vi "Process.vi"(8 "error in":errorcluster, 11 "IPS120":refnum<class "IPS120.lvclass">) -> (0 "error out":errorcluster, 3 "IPS120 out":refnum<class "IPS120.lvclass">)   [LabVIEW 2016, in "IPS120.lvclass"]
doc: "---------------------------------------------------------------\nJKI State Machine Objects™\nhttp://jki.net/state-machine-objects/\nCopyright (C) 2005-2015, JKI <info@jki.net>\nALL RIGHTS RESERVED"
uses:
  IPS120.lvclass
  IPS120/Typedefs/Read System 1 - Enum.ctl
  IPS120/Typedefs/Read System 2 - Enum.ctl
  IPS120/Typedefs/Read Activity - Enum.ctl
  IPS120/Typedefs/Read Switch Heater - Enum.ctl
  IPS120/Typedefs/Read Mode 1 - Enum.ctl
  IPS120/Typedefs/Read Mode 2 - Enum.ctl
  C:/Program Files (x86)/National Instruments/LabVIEW 2016/vi.lib/JKI/JKI SMO/SMO/SMO.lvclass
  <vilib>/JKI/JKI SMO/SMO/Typedefs/Parent Call--Enum.ctl
  <userlib>/LevyLab/Levylab Instruments/SMOs/Instrument/Instrument.lvclass
  <vilib>/JKI/JKI SMO/SMO/SMO.lvclass
  IPS-120.lvlib
panel:
  in  "Tab Control":enum32{"Front Panel", "Error Log"}(tab)
  out "Switch Message":string="Clamped"
  out "Persistent Field (T)":dbl=0.0001 format="%#.5f"
  out "PS Status":bool
  out "system status":T7={"System 1"=enum."Normal", "System 2"=enum."Outside Positive Current Limi", "Activity"=enum."Hold", "Switch Heater"=enum."No Switch Fitted", "Mode 1"=enum."Amps Fast", "Mode 2"=enum."At Rest"}
  out "Current (A)":dbl(knob)=0.0006 scale=-180.0..180.0
  out "Voltage (V) 2":dbl(knob)=-0.0003 caption="Voltage (V)" scale=-10.0..10.0
  out "Sentinel":bool=TRUE
  in  "Remote Mode":bool
  out "Power Supply Field (T)":dbl=0.0001 format="%#.5f"
  out "Voltage (V)":dbl=-0.0003 format="%.5f"
  out "PS Current (A)":dbl=0.0006 format="%.4f"
  out "Magnet Field (T)":dbl(knob) caption="Voltage (V)" scale=-20.0..20.0
  in  "Stop":bool
  out "Switch Time":string="11:11:48"
  in  "PS Heat":bool
  in  "Clamp":bool
  in  "To Set":bool
  in  "To Zero":bool
  in  "Hold":bool
  out "Magnet Activity":string="Clamped"
  out "Target Field Rate (T/min)":dbl=1.0 format="%.5f"
  out "Target Field (T) 2":dbl format="%#.5f"
  in  "Target Rate (T/min)":dbl=0.1 format="%.5f"
  in  "Target Field (T)":dbl format="%#.5f"
  in  "Send to IPS":bool
  out "Error List":T8(array[cluster])
  in  "IPS120 Address":refnum<visa-resource-name>="GPIB1::24::INSTR"
  # "For instructions on how to use the JKI State Machine Objects, examples and video tutorials, visit:\nhttp://jki.net/state-machine-objects/\n\nJKI State Machine Objects™\nhttp://jki.net/state-machine-objects/\nCopyright (C) 2005-2015, JKI <info@jki.net>\nALL RIGHTS RESERVED"
  # "System Status"
  # "Current (A)"
  # "Voltage (V)"
  # "Magnet (T)"
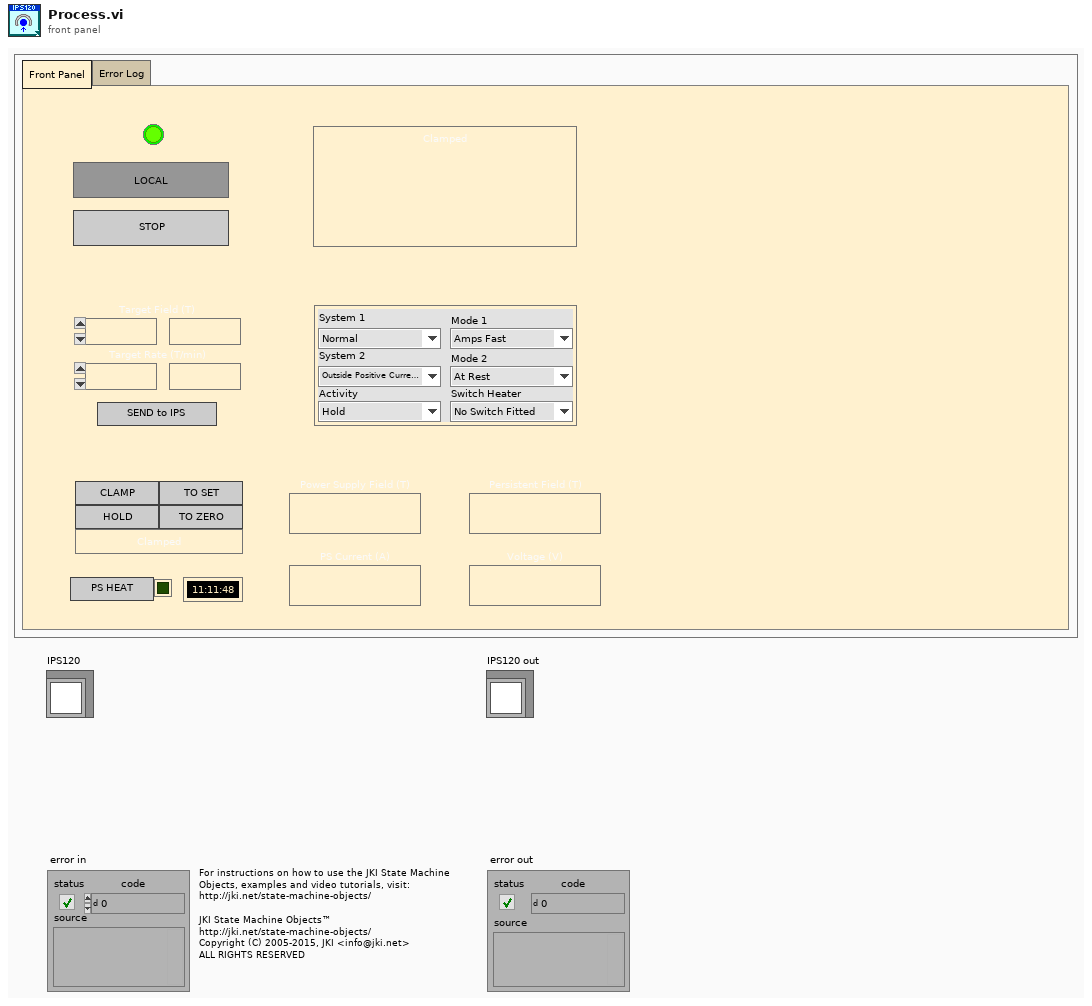
[diagram p1: front panel]
types:
  T1 = typedef "IPS-120.lvlib/Read System 1 - Enum.ctl" = enum16{"Normal", "Quenched", "Over Heated", "Warming Up", "Fault"}
  T2 = typedef "IPS-120.lvlib/Read System 2 - Enum.ctl" = enum16{"Normal", "On Positive Voltage Limit", "On Negative Voltage Limit", "Outside Negative Current Limit", "Outside Positive Current Limi"}
  T3 = typedef "IPS-120.lvlib/Read Activity - Enum.ctl" = enum16{"Hold", "To Set Point", "To Zero", "Clamped"}
  T4 = typedef "IPS-120.lvlib/Read Switch Heater - Enum.ctl" = enum16{"Off Magnet at Zero", "On", "Off Magnet at Field", "Heater Fault", "No Switch Fitted"}
  T5 = typedef "IPS-120.lvlib/Read Mode 1 - Enum.ctl" = enum16{"Amps Fast", "Tesla Fast", "Amps Slow", "Tesla Slow"}
  T6 = typedef "IPS-120.lvlib/Read Mode 2 - Enum.ctl" = enum16{"At Rest", "Sweeping", "Sweep Limiting", "Sweeping & Sweep Limiting"}
  T7 = cluster{"System 1":T1, "System 2":T2, "Activity":T3, "Switch Heater":T4, "Mode 1":T5, "Mode 2":T6}
  T8 = cluster{"time":timestamp, "code":i32, "source":string}[]
  T9 = typedef "SMO.lvclass/Parent Call--Enum.ctl" = enum16{"Allows parent to run", "Does not request parent to run"}
  T10 = enum32{"invalid app kind", "Development System", "Run Time System", "Student Edition", "Embedded LabVIEW", "Evaluation", "Custom"}
  T11 = enum32{"Invalid", "Standard", "Closed", "Hidden", "Minimized", "Maximized"}
  T12 = enum32{"Bad", "Idle", "Run top level", "Running"}
  T13 = cluster{"Core":cluster{"Current VI Reference":refnum<vi>, "Close Panel on Exit?":bool, "error":errorcluster}, "Self Reference":refnum<class "IPS120.lvclass">, "Your string data":string}
  T14 = cluster{"Current VI Reference":refnum<vi>, "Close Panel on Exit?":bool, "error":errorcluster}
  T15 = typedef "SMO.lvclass/Protected Events.ctl" = cluster{"StopProcesses":refnum<user-event>, "AbortProcesses":refnum<user-event>, "Config Changed":refnum<user-event>, "Dependency":refnum<user-event>}
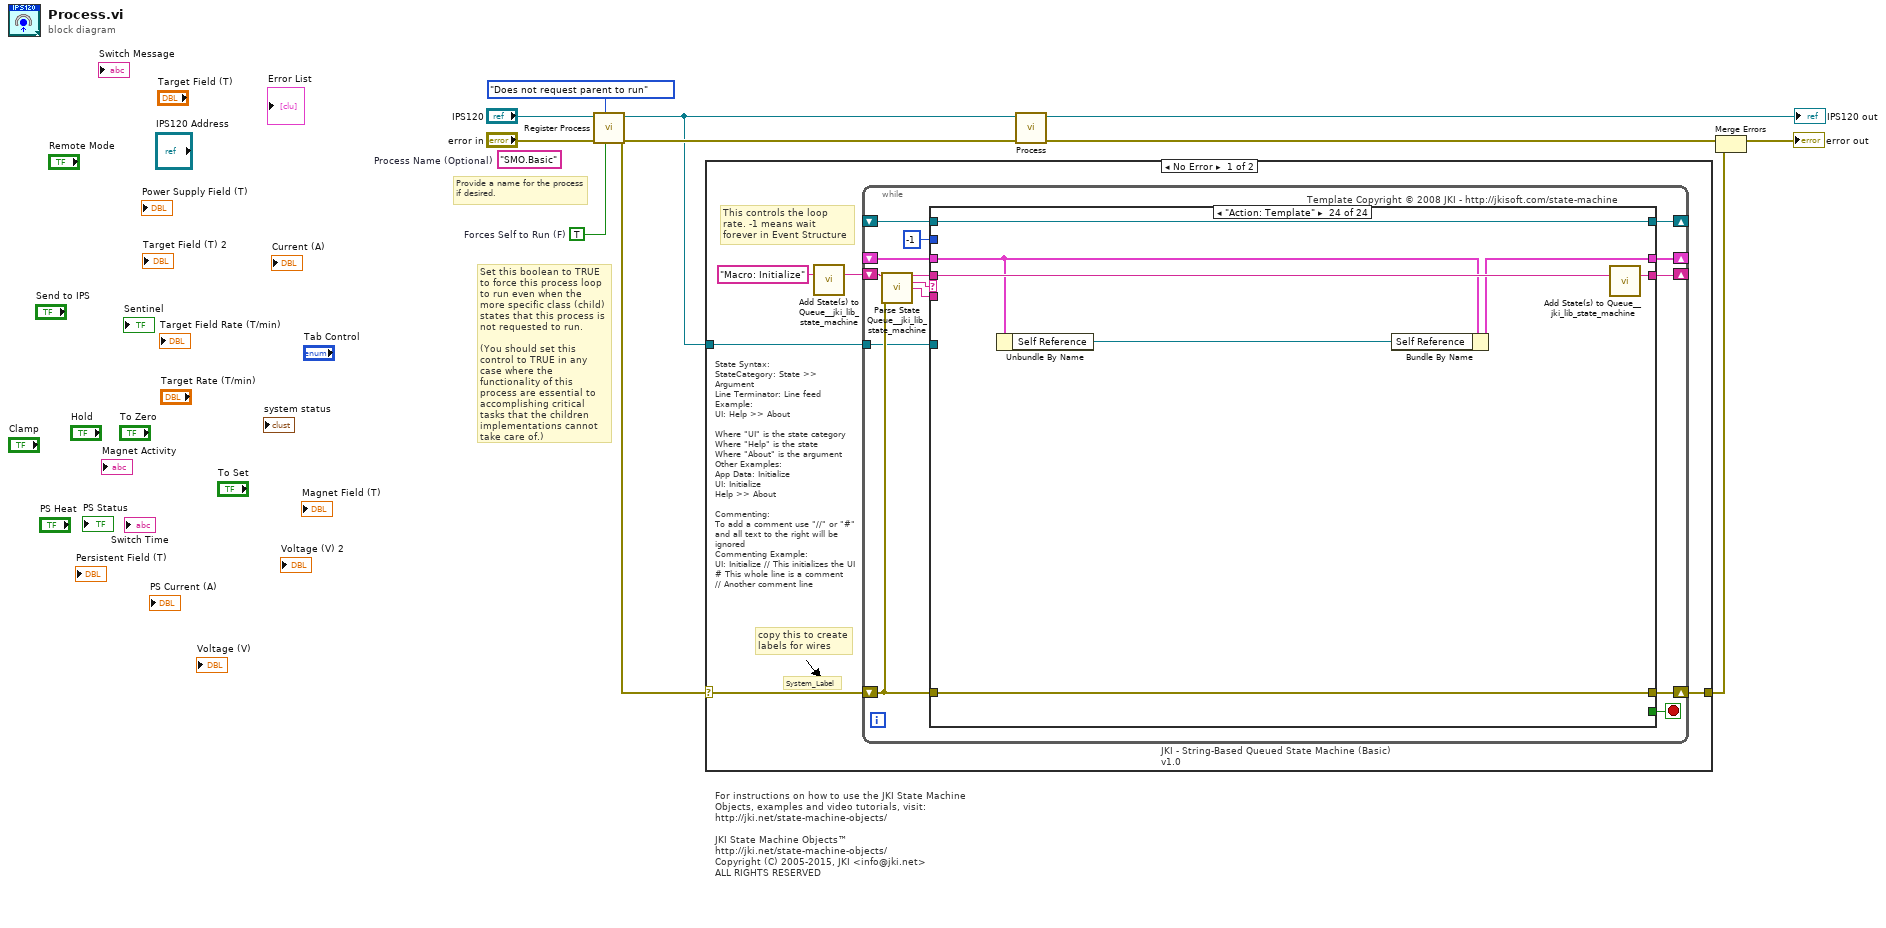
[diagram p0: block diagram]
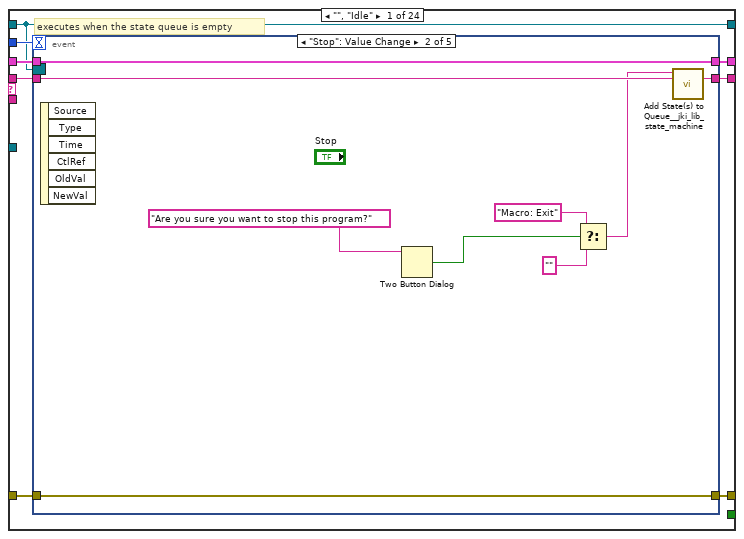
[diagram p2: hidden frame]
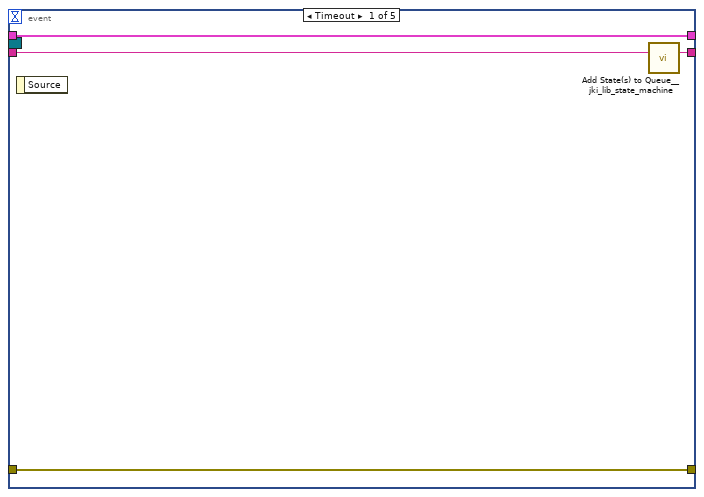
[diagram p3: hidden frame]
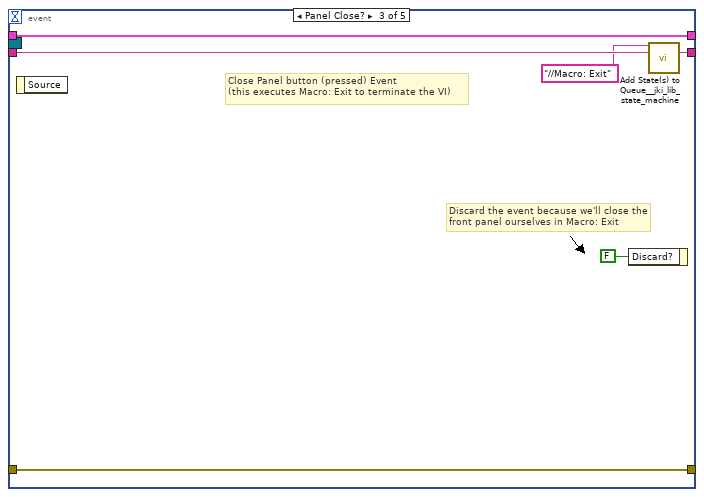
[diagram p4: hidden frame]
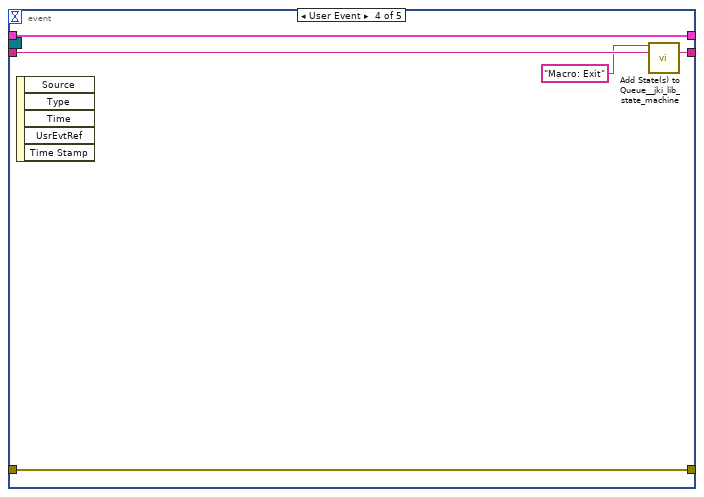
[diagram p5: hidden frame]
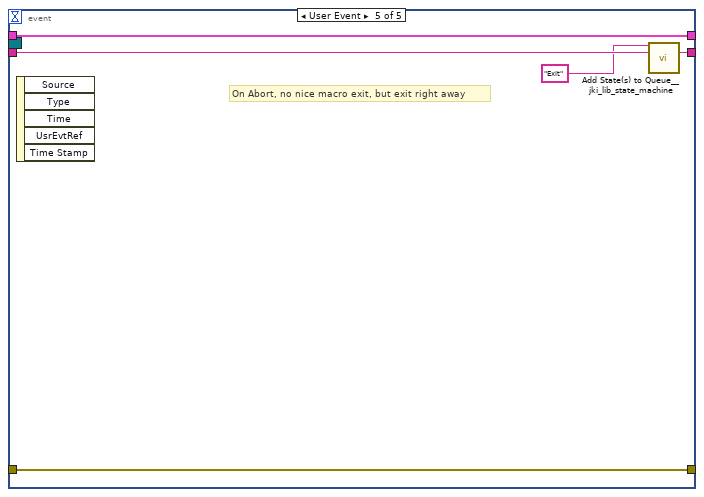
[diagram p6: hidden frame]
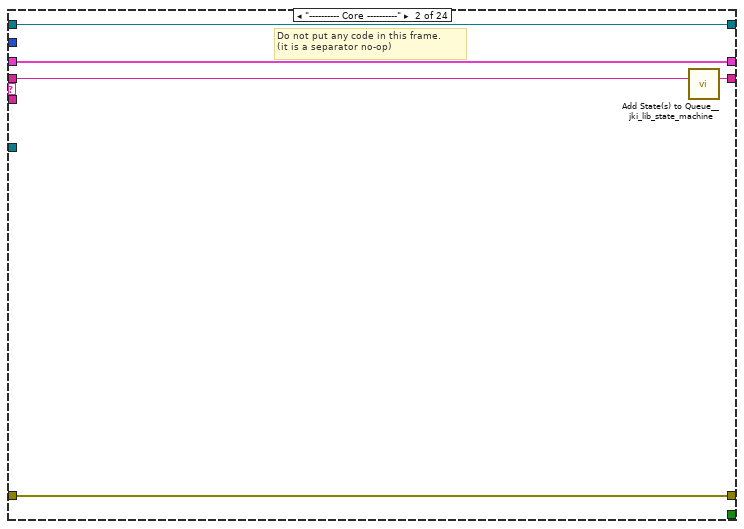
[diagram p7: hidden frame]
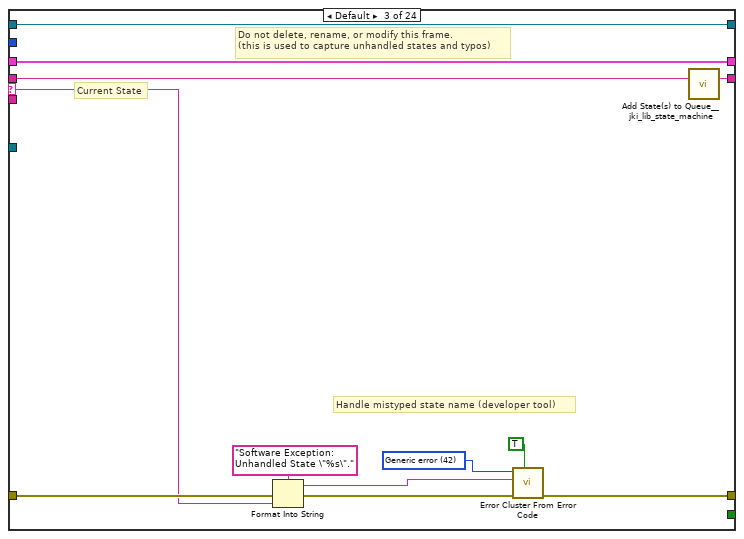
[diagram p8: hidden frame]
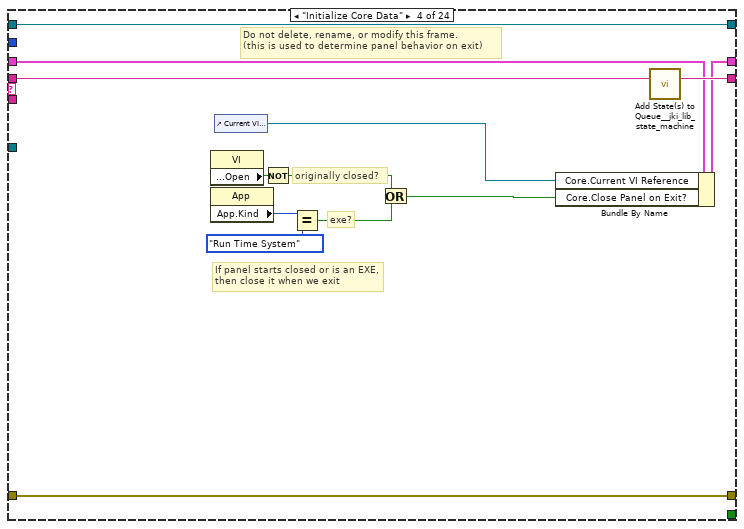
[diagram p9: hidden frame]
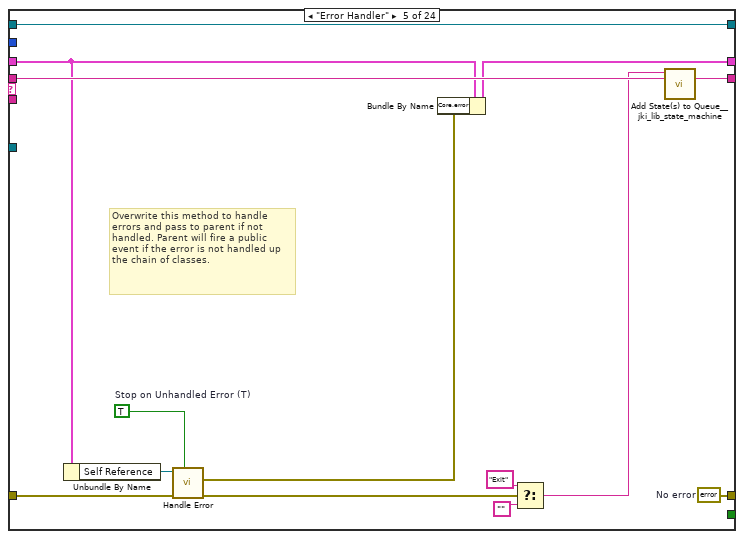
[diagram p10: hidden frame]
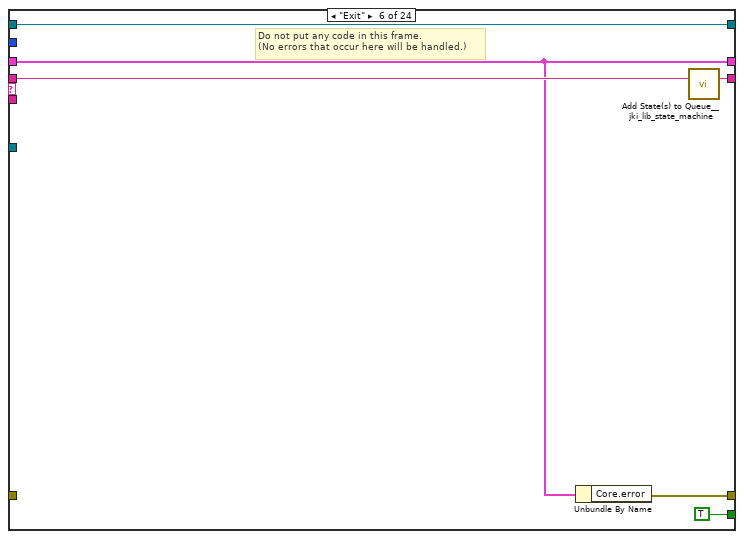
[diagram p11: hidden frame]
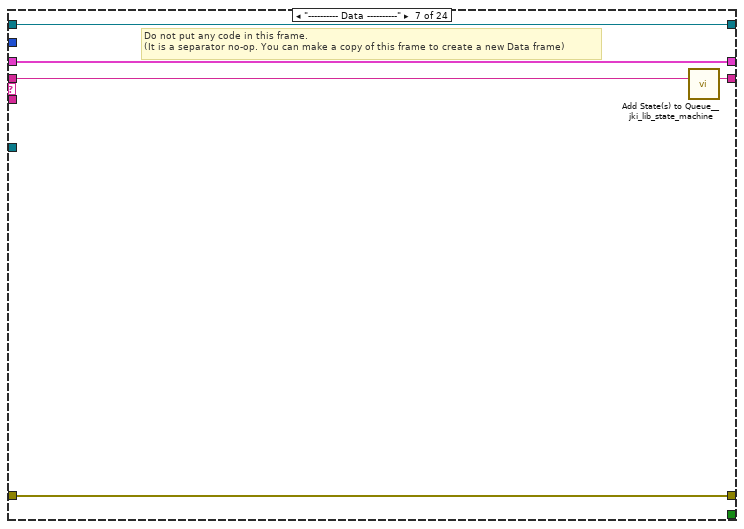
[diagram p12: hidden frame]
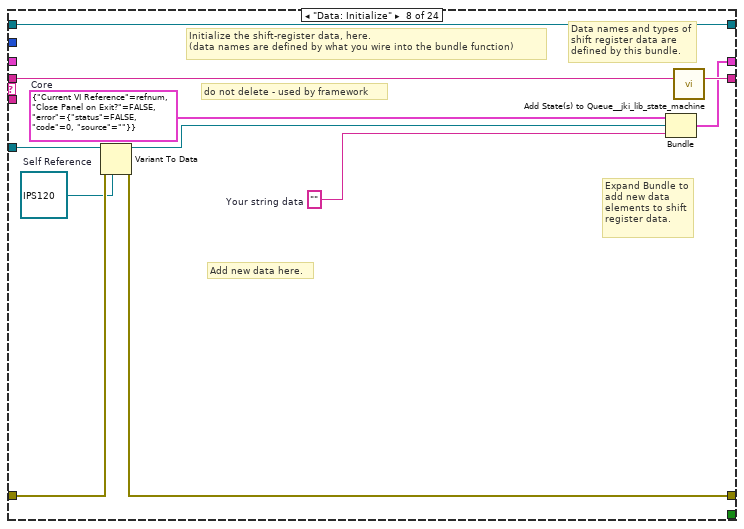
[diagram p13: hidden frame]
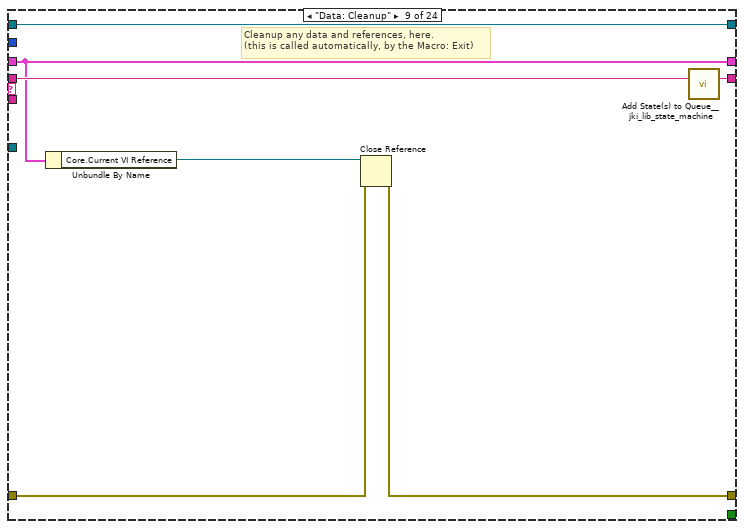
[diagram p14: hidden frame]
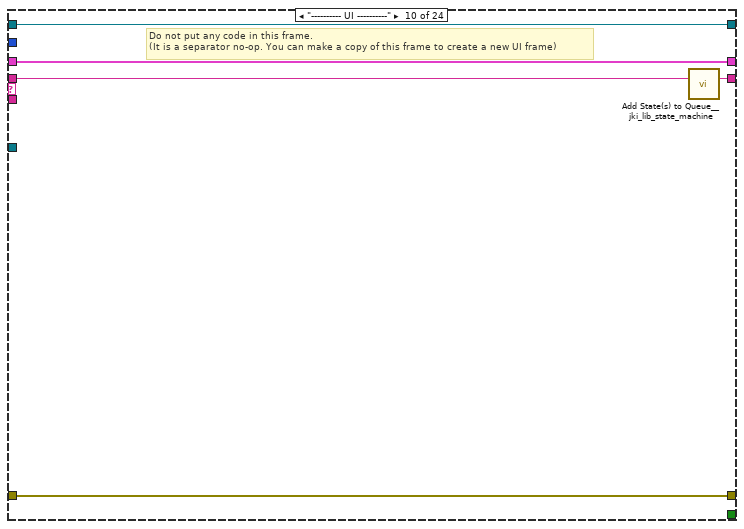
[diagram p15: hidden frame]
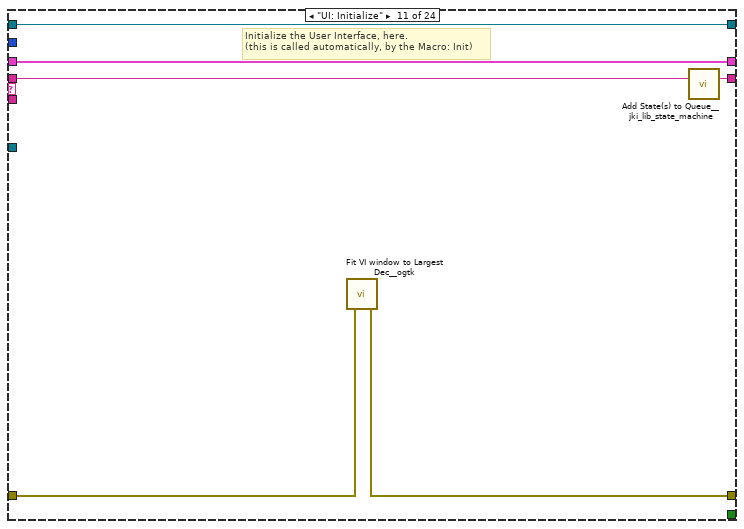
[diagram p16: hidden frame]
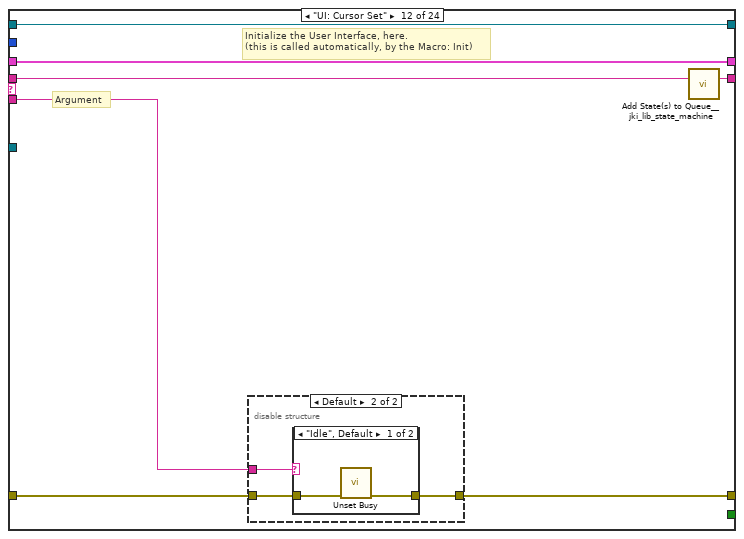
[diagram p17: hidden frame]
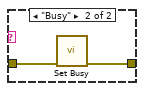
[diagram p19: hidden frame]
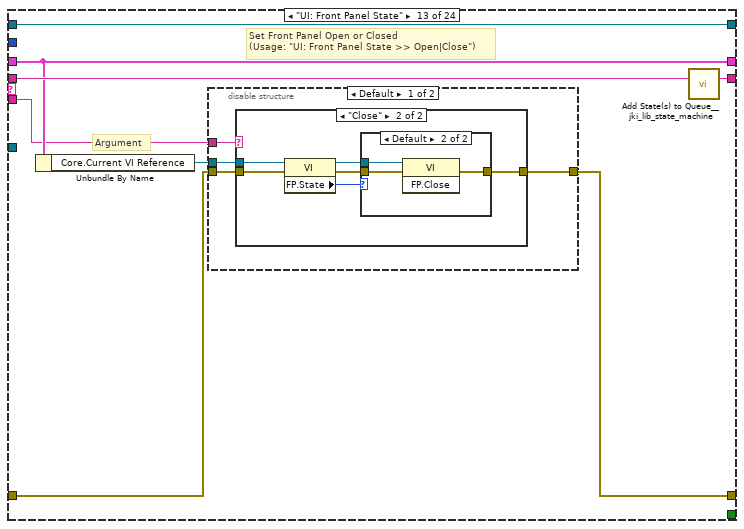
[diagram p20: hidden frame]
diagram:
  w1 = TRUE  # Forces Self to Run (F)
  (unwired) "SMO.Basic"  # Process Name (Optional)
  # "Provide a name for the process\nif desired."
  # "Set this boolean to TRUE to force this process loop to run even when the more specific class (child) states that this process is not requested to run.\n\n(You should set this control to TRUE in any case where the functionality of this process are essential to accomplishing critical tasks that the children implementations cannot take care of.)"
  # "For instructions on how to use the JKI State Machine Objects, examples and video tutorials, visit:\nhttp://jki.net/state-machine-objects/\n\nJKI State Machine Objects™\nhttp://jki.net/state-machine-objects/\nCopyright (C) 2005-2015, JKI <info@jki.net>\nALL RIGHTS RESERVED"
  n1 = call <vilib>:"Register Process.vi"("Forces Self to Run (F)"=w1, "Parent Call"=Parent_Call--Enum."Does not request parent to run", "error in (no error)"="error in", "SMO"="IPS120") -> ("error out"=w7:errorcluster, "SMO out"=w6:refnum<class "IPS120.lvclass">)  [unwired: 6 in]
  n2 = case shown="No Error" w7 {
    selector: w7 -> [w12 w290]
    tunnel: w6 -> [w13 _]
    tunnel: [w11 w290] -> w3
    frame No Error {
      # "State Syntax:\nStateCategory: State >> Argument\nLine Terminator: Line feed\nExample:\nUI: Help >> About\n\nWhere \"UI\" is the state category\nWhere \"Help\" is the state\nWhere \"About\" is the argument\nOther Examples:\nApp Data: Initialize\nUI: Initialize\nHelp >> About\n\nCommenting:\nTo add a comment use \"//\" or \"#\" and all text to the right will be ignored\nCommenting Example:\nUI: Initialize // This initializes the UI\n# This whole line is a comment\n// Another comment line"
      # "copy this to create labels for wires"
      # "This controls the loop rate. -1 means wait forever in Event Structure"
      # "System_Label"
      n3 = call <vilib>:"Add State(s) to Queue__jki_lib_state_machine.vi"("State(s) in (\"\")"="Macro: Initialize") -> ("States Out"=w15:string)  [unwired: 14 in]
      n4 = while "JKI - String-Based Queued State Machine (Basic) v1.0" {
        shift-right: [w22] -> _
        shift-left: _ -> [w21]
        shift-right: [w25] -> w11
        shift-left: w12 -> [w19]
        shift-right: [w24] -> _
        shift-left: w15 -> [w26]
        tunnel: w13 -> [w18]
        shift-right: [w17] -> _
        shift-left: _ -> [w16]
        stop <- w23 stop-if-true
        # "Template Copyright © 2008 JKI - http://jkisoft.com/state-machine"
        n5 = call <vilib>:"Parse State Queue__jki_lib_state_machine.vi"("State Queue"=w26, "Error In (no error)"=w19) -> ("Remaining States"=w28:string, "Current State"=w29:string, "Arguments"=w27:string)  [unwired: 11 in]
        n6 = case shown="\"Action: Template\"" w29 {
          selector: w29 -> [_ _ w73 _ _ _ _ _ _ _ _ _ _ _ _ _ _ _ _ _ _ _ _ _]
          tunnel: w28 -> [w37 w71 w77 w96 w110 w116 w121 w132 w139 w144 w150 w157 w173 w205 w219 w233 w238 w249 w256 w261 w271 w277 w282 w289]
          tunnel: w27 -> [_ _ _ _ _ _ _ _ _ _ _ w151 w167 _ _ _ _ _ _ _ _ _ _ _]
          tunnel: w21 -> [w35 w68 w75 w87 w104 w112 w118 _ w134 w141 w148 w155 w169 w202 w215 w224 w235 w246 w252 w258 w269 w275 w280 w285]
          tunnel: [w34 w69 w79 w93 w105 w111 w119 w127 w135 w142 w145 w152 w170 w203 w217 w231 w236 w240 w250 w259 w264 w273 w278 w286] -> w25
          tunnel: w19 -> [w33 w69 w78 w93 w106 _ w119 w128 w136 w142 w146 w153 w171 w203 w217 w231 w236 w241 w251 w259 w265 w273 w278 w286]
          tunnel: [w36 w70 w76 w95 w109 w115 w120 w131 w138 w143 w149 w156 w172 w204 w218 w232 w237 w248 w255 w260 w270 w276 w281 w288] -> w24
          tunnel: [_ _ _ _ _ TRUE _ _ _ _ _ _ _ _ _ _ _ _ _ _ _ _ _ _] -> w23
          tunnel: [w32 w68 w75 w94 w103 w112 w118 w130 w134 w141 w148 w155 w169 w202 w215 w224 w235 w246 w252 w258 w269 w275 w280 w284] -> w22
          tunnel: -1 ("Timeout") -> [w31 _ _ _ _ _ _ _ _ _ _ _ _ _ _ _ _ _ _ _ _ _ _ _]
          tunnel: w18 -> [_ _ _ _ _ _ _ w125 _ _ _ _ _ _ _ _ _ _ _ _ _ _ _ _]
          tunnel: [w30 w67 w72 w84 w108 w113 w117 w123 w133 w140 w147 w154 w166 w201 w216 w225 w234 w247 w254 w257 w268 w274 w279 w287] -> w17
          tunnel: w16 -> [w30 w67 w72 w84 w108 w113 w117 w123 w133 w140 w147 w154 w166 w201 w216 w225 w234 w247 w254 w257 _ w274 w279 w287]
          frame "", "Idle" {
            # "executes when the state queue is empty"
            n7 = event shown="[1] \"Stop\": Value Change" {
              selector: w30 -> [_ _ _ _ _]
              dyn-events: _ -> [_ _ _ _ _]
              timeout: w31 -> [_ _ _ _ _]
              tunnel: w37 -> [w41 w50 w56 w61 w66]
              tunnel: [w40 w49 w55 w60 w65] -> w36
              tunnel: w35 -> [w39 w48 w53 w58 w63]
              tunnel: [w38 w47 w54 w59 w64] -> w34
              tunnel: w33 -> [w38 w47 w54 w59 w64]
              tunnel: [w39 w48 w53 w58 w63] -> w32
              event Timeout {
                n8 = event-data() -> ()  [unwired: 1 in, 1 out]
                n9 = call <vilib>:"Add State(s) to Queue__jki_lib_state_machine.vi"("State(s) in (\"\")"=w41) -> ("States Out"=w40:string)  [unwired: 14 in]
              }
              event "Stop": Value Change {
                n10 = event-data() -> ()  [unwired: 1 in, 6 out]
                n11 = Two Button Dialog(message="Are you sure you want to stop this program?") -> (T button?=w46:bool)  [unwired: 2 in]
                n12 = Select(t="Macro: Exit", s=w46, f="") -> (s? t:f=w42:string)
                n13 = call <vilib>:"Add State(s) to Queue__jki_lib_state_machine.vi"("State(s) in Front (\"\")"=w42, "State(s) in (\"\")"=w50) -> ("States Out"=w49:string)  [unwired: 13 in]
              }
              event Panel Close? {
                # "Discard the event because we'll close the front panel ourselves in Macro: Exit"
                # "Close Panel button (pressed) Event\n(this executes Macro: Exit to terminate the VI)"
                n14 = event-data() -> ()  [unwired: 1 in, 1 out]
                n15 = event-data("Discard?"=FALSE) -> ()  [unwired: 1 in, 1 out]
                n16 = call <vilib>:"Add State(s) to Queue__jki_lib_state_machine.vi"("State(s) in Front (\"\")"="//Macro: Exit", "State(s) in (\"\")"=w56) -> ("States Out"=w55:string)  [unwired: 13 in]
              }
              event User Event {
                n17 = event-data() -> ()  [unwired: 1 in, 5 out]
                n18 = call <vilib>:"Add State(s) to Queue__jki_lib_state_machine.vi"("State(s) in Front (\"\")"="Macro: Exit", "State(s) in (\"\")"=w61) -> ("States Out"=w60:string)  [unwired: 13 in]
              }
              event User Event {
                # "On Abort, no nice macro exit, but exit right away"
                n19 = event-data() -> ()  [unwired: 1 in, 5 out]
                n20 = call <vilib>:"Add State(s) to Queue__jki_lib_state_machine.vi"("State(s) in Front (\"\")"="Exit", "State(s) in (\"\")"=w66) -> ("States Out"=w65:string)  [unwired: 13 in]
              }
            }
          }
          frame "---------- Core ----------" {
            # "Do not put any code in this frame.\n(it is a separator no-op)"
            n21 = call <vilib>:"Add State(s) to Queue__jki_lib_state_machine.vi"("State(s) in (\"\")"=w71) -> ("States Out"=w70:string)  [unwired: 14 in]
          }
          frame Default {
            w82 = 42 items=["No error", "Argument error", "Memory is full", "Out of zone", "End of file", "File already open", "Generic file I/O error", "File not found", "File permission error", "Disk is full", "Duplicate path", "Too many files open", "System feature not enabled", "Resource file not found", "Cannot add resource", "Resource not found", "Image not found", "Image memory error", "Pen does not exist", "Config type invalid", "Config token not found", "Config parse error", "Config memory error", "Bad external code format", "Bad external code offset", "External code not present", "Null window", "Destroy window error", "Null menu", "Print aborted", "Bad print record", "Print driver error", "Windows error during printing", "Memory error during printing", "Print dialog error", "Generic print error", "Invalid device refnum", "Device not found", "Device parameter error", "Device unit error", "Cannot open device", "Device call aborted", "Generic error", "Cancelled by user", "Object ID too low", "Object ID too high", "Object not in heap", "Unknown heap", "Unknown object (invalid DefProc)", "Unknown object (DefProc not in table)", "Message out of range", "Invalid (null) method", "Unknown message", "Manager call not supported", "Bad address", "Network operation in progress", "Network operation timed out", "Connection is busy", "Network attribute not supported", "Network error", "Address in use", "System out of memory", "Connection aborted", "Connection refused", "Not connected", "Already connected", "Connection closed", "Initialization error (interapplication manager)", "Bad occurrence", "Wait on unbound occurrence handler", "Occurrence queue overflow", "Datalog type conflict", "Unused", "Unrecognized type (interapplication manager)", "Memory corrupt", "Failed to make temporary DLL", "Old CIN version", "Drag socket not found", "Failed to load drop-object", "Failed to register OLE object", "Failed to release OLE object", "Format specifier type mismatch", "Unknown format specifier", "Too few format specifiers", "Too many format specifiers", "Scan failed", "Newer CIN version", "Error converting to variant", "Runtime menu error", "Password tampered", "Variant attribute not found", "Incompatible variant data type", "Event data is not available", "Event Store is not present", "Occurrence is not found", "Event Queue is not created", "Event info is not available", "Refnum passed is NULL", "Error retrieving Class GUID", "Error retrieving CoClass GUID", "Error retrieving TypeLib GUID.", "Bad built application magic bytes.", "Specific driver is different from the specific driver associated with the Logical Name.", "There is no session opened to the class driver.", "Max Error", "MAX - Error with config objects", "MAX - Error loading configuration", "MAX - Group not supported"]
            # "Current State"
            # "Do not delete, rename, or modify this frame.\n(this is used to capture unhandled states and typos)"
            # "Handle mistyped state name (developer tool)"
            n22 = Format Into String(format string="Software Exception: Unhandled State \"%s\"." ("message"), error in=w78, w73) -> (resulting string=w81:string, error out=w80:errorcluster)  [unwired: 1 in]
            n23 = call <vilib>:"Error Cluster From Error Code.vi"("show call chain? (False)"=TRUE, "error in (no error)"=w80, "error message (\"\")"=w81, "error code (0)"=w82) -> ("error out"=w79:errorcluster)  [unwired: 5 in]
            n24 = call <vilib>:"Add State(s) to Queue__jki_lib_state_machine.vi"("State(s) in (\"\")"=w77) -> ("States Out"=w76:string)  [unwired: 14 in]
          }
          frame "Initialize Core Data" {
            # "Do not delete, rename, or modify this frame.\n(this is used to determine panel behavior on exit)"
            # "originally closed?"
            # "exe?"
            # "If panel starts closed or is an EXE, then close it when we exit"
            n25 = property class="VI"() -> ("Front Panel.Open"=w92:bool)  [unwired: 2 in, 2 out]
            n26 = property class="App"() -> ("App.Kind"=w91:T10)  [unwired: 2 in, 2 out]
            n27 = control-ref of="Current VI Reference"() -> (w85:refnum<vi>)
            n28 = Not(x=w92) -> (.not. x?=w89:bool)
            n29 = Equal?(x=w91, y=T10."Run Time System" ("Application:Kind")) -> (x = y?=w88:bool)
            n30 = Or(x=w89, y=w88) -> (x .or. y?=w86:bool)
            n31 = Bundle By Name(cluster=w87, "Core.Current VI Reference"=w85, "Core.Close Panel on Exit?"=w86) -> (w94:T13)
            n32 = call <vilib>:"Add State(s) to Queue__jki_lib_state_machine.vi"("State(s) in (\"\")"=w96) -> ("States Out"=w95:string)  [unwired: 14 in]
          }
          frame "Error Handler" {
            w97 = TRUE  # Stop on Unhandled Error (T)
            w105 = errorcluster {"status"=FALSE, "code"=0, "source"=""}  # No error
            # "Overwrite this method to handle errors and pass to parent if not handled. Parent will fire a public event if the error is not handled up the chain of classes."
            n33 = Unbundle By Name(w104) -> ("Self Reference"=w107:refnum<class "IPS120.lvclass">)
            n34 = call-dynamic "Handle Error.vi"("Stop on Unhandled Error (T)"=w97, "error in"=w106, "Instrument"=w107) -> ("handling error"=w98:errorcluster, "Unhandled error"=w101:errorcluster)  [unwired: 6 in, 1 out]
            n35 = Bundle By Name(cluster=w104, "Core.error"=w101) -> (w103:T13)
            n36 = Select(t="Exit", s=w98, f="") -> (s? t:f=w102:string)
            n37 = call <vilib>:"Add State(s) to Queue__jki_lib_state_machine.vi"("State(s) in Front (\"\")"=w102, "State(s) in (\"\")"=w110) -> ("States Out"=w109:string)  [unwired: 13 in]
          }
          frame "Exit" {
            # "Do not put any code in this frame.\n(No errors that occur here will be handled.)"
            n38 = Unbundle By Name(w112) -> ("Core.error"=w111:errorcluster)
            n39 = call <vilib>:"Add State(s) to Queue__jki_lib_state_machine.vi"("State(s) in (\"\")"=w116) -> ("States Out"=w115:string)  [unwired: 14 in]
          }
          frame "---------- Data ----------" {
            # "Do not put any code in this frame.\n(It is a separator no-op. You can make a copy of this frame to create a new Data frame)"
            n40 = call <vilib>:"Add State(s) to Queue__jki_lib_state_machine.vi"("State(s) in (\"\")"=w121) -> ("States Out"=w120:string)  [unwired: 14 in]
          }
          frame "Data: Initialize" {
            w122 = T14 {"Current VI Reference"=refnum, "Close Panel on Exit?"=FALSE, "error"={"status"=FALSE, "code"=0, "source"=""}}  # Core
            w126 = refnum<class "IPS120.lvclass"> refnum  # Self Reference
            w129 = ""  # Your string data
            # "do not delete - used by framework"
            # "Expand Bundle to add new data elements to shift register data."
            # "Add new data here."
            # "Data names and types of shift register data are defined by this bundle."
            # "Initialize the shift-register data, here.\n(data names are defined by what you wire into the bundle function)"
            n41 = Variant To Data(error in=w128, type=w126, Variant=w125) -> (data=w124:refnum<class "IPS120.lvclass">, error out=w127:errorcluster)
            n42 = Bundle("Core"=w122, "Self Reference"=w124, "Your string data"=w129) -> (w130:T13)  [unwired: 1 in]
            n43 = call <vilib>:"Add State(s) to Queue__jki_lib_state_machine.vi"("State(s) in (\"\")"=w132) -> ("States Out"=w131:string)  [unwired: 14 in]
          }
          frame "Data: Cleanup" {
            # "Cleanup any data and references, here.\n(this is called automatically, by the Macro: Exit)"
            n44 = Unbundle By Name(w134) -> ("Core.Current VI Reference"=w137:refnum<vi>)
            n45 = Close Reference(reference=w137, error in (no error)=w136) -> (error out=w135:errorcluster)
            n46 = call <vilib>:"Add State(s) to Queue__jki_lib_state_machine.vi"("State(s) in (\"\")"=w139) -> ("States Out"=w138:string)  [unwired: 14 in]
          }
          frame "---------- UI ----------" {
            # "Do not put any code in this frame.\n(It is a separator no-op. You can make a copy of this frame to create a new UI frame)"
            n47 = call <vilib>:"Add State(s) to Queue__jki_lib_state_machine.vi"("State(s) in (\"\")"=w144) -> ("States Out"=w143:string)  [unwired: 14 in]
          }
          frame "UI: Initialize" {
            # "Initialize the User Interface, here.\n(this is called automatically, by the Macro: Init)"
            n48 = call <userlib>:"Fit VI window to Largest Dec__ogtk.vi"("error in (no error)"=w146) -> ("error out"=w145:errorcluster)  [unwired: 5 in, 1 out]
            n49 = call <vilib>:"Add State(s) to Queue__jki_lib_state_machine.vi"("State(s) in (\"\")"=w150) -> ("States Out"=w149:string)  [unwired: 14 in]
          }
          frame "UI: Cursor Set" {
            # "Argument"
            # "Initialize the User Interface, here.\n(this is called automatically, by the Macro: Init)"
            n50 = disable-structure shown="Default" {
              disable-tunnel: w153 -> [w158 w161]
              disable-tunnel: [w158 w160] -> w152
              disable-tunnel: w151 -> [_ w159]
              frame condition #0 {
              }
              frame condition #1 (active) {
                n51 = case shown="\"Idle\", Default" w159 {
                  tunnel: w161 -> [w163 w165]
                  tunnel: [w162 w164] -> w160
                  frame "Idle", Default {
                    n52 = call <vilib>:"Unset Busy.vi"("error in (no error)"=w163) -> ("error out"=w162:errorcluster)  [unwired: 10 in]
                  }
                  frame "Busy" {
                    n53 = call <vilib>:"Set Busy.vi"("error in (no error)"=w165) -> ("error out"=w164:errorcluster)  [unwired: 9 in, 1 out]
                  }
                }
              }
            }
            n54 = call <vilib>:"Add State(s) to Queue__jki_lib_state_machine.vi"("State(s) in (\"\")"=w157) -> ("States Out"=w156:string)  [unwired: 14 in]
          }
          frame "UI: Front Panel State" {
            # "Argument"
            # "Set Front Panel Open or Closed\n(Usage: \"UI: Front Panel State >> Open|Close\")"
            n55 = Unbundle By Name(w169) -> ("Core.Current VI Reference"=w168:refnum<vi>)
            n56 = disable-structure shown="Default" {
              disable-tunnel: w171 -> [w177 w200]
              disable-tunnel: [w176 w200] -> w170
              disable-tunnel: w168 -> [w175 _]
              disable-tunnel: w167 -> [w174 _]
              frame condition #0 (active) {
                n57 = case shown="\"Close\"" w174 {
                  tunnel: w177 -> [w181 w194]
                  tunnel: [w183 w195] -> w176
                  tunnel: w175 -> [w182 w192]
                  frame "Open", Default {
                    n58 = property class="VI"(reference=w182, error in=w181) -> (reference out=w179:refnum<vi>, error out=w180:errorcluster, "FP.State"=w178:T11)
                    n59 = case shown="\"Closed\"" w178 {
                      tunnel: [w186 w189] -> w183
                      tunnel: w180 -> [w185 w189]
                      tunnel: w179 -> [w184 _]
                      frame "Closed" {
                        n60 = invoke class="VI" method="FP.Open"(reference=w184, error in=w185, "Activate"=TRUE, "State"=T11."Standard") -> (error out=w186:errorcluster)  [unwired: 1 in, 4 out]
                      }
                      frame Default {
                      }
                    }
                  }
                  frame "Close" {
                    n61 = property class="VI"(reference=w192, error in=w194) -> (reference out=w191:refnum<vi>, error out=w193:errorcluster, "FP.State"=w190:T11)
                    n62 = case shown="Default" w190 {
                      tunnel: [w196 w199] -> w195
                      tunnel: w193 -> [w196 w198]
                      tunnel: w191 -> [_ w197]
                      frame "Invalid", "Closed" {
                      }
                      frame Default {
                        n63 = invoke class="VI" method="FP.Close"(reference=w197, error in=w198) -> (error out=w199:errorcluster)  [unwired: 1 in, 2 out]
                      }
                    }
                  }
                }
              }
              frame condition #1 {
              }
            }
            n64 = call <vilib>:"Add State(s) to Queue__jki_lib_state_machine.vi"("State(s) in (\"\")"=w173) -> ("States Out"=w172:string)  [unwired: 14 in]
          }
          frame "---------- Macro ----------" {
            # "Do not put any code in this frame.\n(It is a separator no-op. You can make a copy of this frame to create a new Macro frame)"
            n65 = call <vilib>:"Add State(s) to Queue__jki_lib_state_machine.vi"("State(s) in (\"\")"=w205) -> ("States Out"=w204:string)  [unwired: 14 in]
          }
          frame "Macro: Initialize" {
            w210 = "UI: Initialize\nUI: Front Panel State >> Open"  # UI: Initialize UI: Front Panel State >> Open
            w206 = "Process: Sync"
            # "Initialization Macro\n(This is called once, when the VI starts)"
            n66 = control-ref of="This VI"() -> (w208:refnum<vi>)
            n67 = property class="VI"(reference=w208) -> ("Exec.State"=w207:T12)  [unwired: 1 in, 2 out]
            n68 = Equal?(x=w207, y=T12."Run top level") -> (x = y?=w213:bool)
            n69 = Select(t=w206, s=w213, f="") -> ()  [unwired: 1 out]
            n70 = call <vilib>:"Add State(s) to Queue__jki_lib_state_machine.vi"("State(s) in Front (\"\")"="Data: Initialize\nInitialize Core Data\nEvents: Register", "State(s) in (\"\")"=w206, "State(s) at Back (\"\")"=w210) -> ("States Out"=w209:string)  [unwired: 12 in]
            n71 = call <vilib>:"Add State(s) to Queue__jki_lib_state_machine.vi"("State(s) in Front (\"\")"=w209, "State(s) in (\"\")"=w219) -> ("States Out"=w218:string)  [unwired: 13 in]
          }
          frame "Macro: Exit" {
            # "Exit Macro\n(This is called once, when the VI exits)"
            n72 = Unbundle By Name(w224) -> ("Core.Close Panel on Exit?"=w230:bool)
            n73 = Select(t="UI: Front Panel State >> Close", s=w230, f="") -> (s? t:f=w227:string)
            n74 = call <vilib>:"Add State(s) to Queue__jki_lib_state_machine.vi"("State(s) in Front (\"\")"="Data: Cleanup\nEvents: Unregister\nProcess: Self Terminate", "State(s) in (\"\")"="Process: Sync", "State(s) at Back (\"\")"="Exit") -> ("States Out"=w221:string)  [unwired: 12 in]
            n75 = call <vilib>:"Add State(s) to Queue__jki_lib_state_machine.vi"("State(s) in (\"\")"=w227, "State(s) at Back (\"\")"=w221) -> ("States Out"=w226:string)  [unwired: 13 in]
            n76 = call <vilib>:"Add State(s) to Queue__jki_lib_state_machine.vi"("State(s) in Front (\"\")"=w226, "State(s) in (\"\")"=w233) -> ("States Out"=w232:string)  [unwired: 13 in]
          }
          frame "---------- Process ----------" {
            # "Template Separator\n(You can make a copy of, or modify, this frame)"
            n77 = call <vilib>:"Add State(s) to Queue__jki_lib_state_machine.vi"("State(s) in (\"\")"=w238) -> ("States Out"=w237:string)  [unwired: 14 in]
          }
          frame "Process: Sync" {
            n78 = Unbundle By Name(w246) -> ("Self Reference"=w242:refnum<class "IPS120.lvclass">)
            n79 = call <vilib>:"WaitOnProcessSync.vi"("error in (no error)"=w241, "SMO"=w242) -> ("error out"=w240:errorcluster, "Don't run?"=w245:bool)  [unwired: 7 in, 1 out]
            n80 = Select(t="Data: Cleanup\nEvents: Unregister\nExit", s=w245, f="") -> (s? t:f=w239:string)
            n81 = call <vilib>:"Add State(s) to Queue__jki_lib_state_machine.vi"("State(s) in Front (\"\")"=w239, "State(s) in (\"\")"=w249) -> ("States Out"=w248:string)  [unwired: 13 in]
          }
          frame "Process: Self Terminate" {
            n82 = Unbundle By Name(w252) -> ("Self Reference"=w253:refnum<class "IPS120.lvclass">)
            n83 = call <vilib>:"SelfTerminate.vi"("error in (no error)"=w251, "SMO in"=w253) -> ("error out"=w250:errorcluster)  [unwired: 8 in, 1 out]
            n84 = call <vilib>:"Add State(s) to Queue__jki_lib_state_machine.vi"("State(s) in (\"\")"=w256) -> ("States Out"=w255:string)  [unwired: 14 in]
          }
          frame "---------- Events ----------" {
            # "Template Separator\n(You can make a copy of, or modify, this frame)"
            n85 = call <vilib>:"Add State(s) to Queue__jki_lib_state_machine.vi"("State(s) in (\"\")"=w261) -> ("States Out"=w260:string)  [unwired: 14 in]
          }
          frame "Events: Register" {
            # "Expand to add\nmore events"
            n86 = Unbundle By Name(w269) -> ("Self Reference"=w266:refnum<class "IPS120.lvclass">)
            n87 = call <vilib>:"GetProtectedEvents.vi"("SMO"=w266) -> ("error out"=w262:errorcluster, "SMO Protected Events"=w267:T15)  [unwired: 8 in, 1 out]
            n88 = register-events(w267) -> (reference out=w268:refnum<event-registration>, error out=w263:errorcluster)  [unwired: 2 in]
            n89 = Merge Errors(w265, w263, w262) -> (w264:errorcluster)
            n90 = call <vilib>:"Add State(s) to Queue__jki_lib_state_machine.vi"("State(s) in (\"\")"=w271) -> ("States Out"=w270:string)  [unwired: 14 in]
          }
          frame "Events: Unregister" {
            n91 = Unregister For Events(event registration refnum=w274, error in=w273) -> (error out=w272:errorcluster)
            n92 = call <vilib>:"Clear Errors.vi"("error in (no error)"=w272) -> ()  [unwired: 5 in, 2 out]
            n93 = call <vilib>:"Add State(s) to Queue__jki_lib_state_machine.vi"("State(s) in (\"\")"=w277) -> ("States Out"=w276:string)  [unwired: 14 in]
          }
          frame "---------- Action ----------" {
            n94 = call <vilib>:"Add State(s) to Queue__jki_lib_state_machine.vi"("State(s) in (\"\")"=w282) -> ("States Out"=w281:string)  [unwired: 14 in]
          }
          frame "Action: Template" {
            n95 = Unbundle By Name(w285) -> ("Self Reference"=w283:refnum<class "IPS120.lvclass">)
            n96 = Bundle By Name(cluster=w285, "Self Reference"=w283) -> (w284:T13)
            n97 = call <vilib>:"Add State(s) to Queue__jki_lib_state_machine.vi"("State(s) in (\"\")"=w289) -> ("States Out"=w288:string)  [unwired: 14 in]
          }
        }
      }
    }
    frame Error {
    }
  }
  n98 = call-parent "Process.vi"("error in"=w7, "Instrument"=w6) -> ("error out"=w4:errorcluster, "Instrument out"=→"IPS120 out":refnum<class "IPS120.lvclass">)  [unwired: 8 in]
  n99 = Merge Errors(w4, w3) -> (→"error out":errorcluster)
